vi "Create Event.vi"(8 "error in":errorcluster, 11 "SEQ in":refnum<class "SEQ.lvclass">) -> (0 "error out":errorcluster, 2 "MSG Event Reg":refnum<event-registration>, 3 "SEQ out":refnum<class "SEQ.lvclass">)   [LabVIEW 2014]
uses:
  SEQ.lvclass
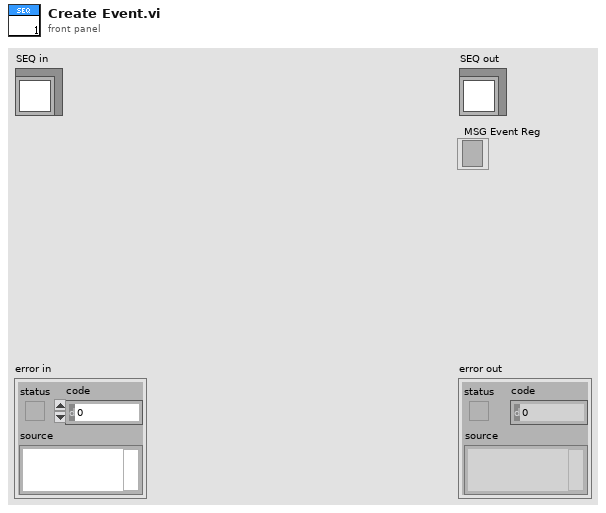
[diagram p1: front panel]
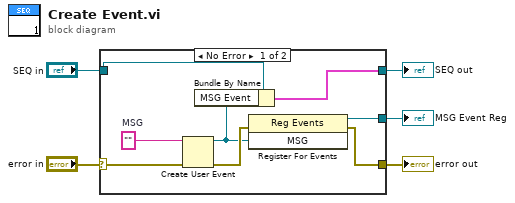
[diagram p0: block diagram]
diagram:
  n1 = case shown="No Error" "error in" {
    selector: "error in" -> [w12 w15]
    tunnel: [w10 w15] -> w4
    tunnel: [w6 w14] -> w2
    tunnel: "SEQ in" -> [w9 w14]
    tunnel: [w7 _] -> w1
    frame No Error {
      w13 = ""  # MSG
      n2 = Create User Event(user event datatype=w13, error in=w12) -> (user event=w8:refnum<user-event>, error out=w11:errorcluster)
      n3 = Bundle By Name(cluster=w9, "MSG Event"=w8) -> (w6:cluster{})
      n4 = register-events(error in=w11, w8) -> (reference out=w7:refnum<event-registration>, error out=w10:errorcluster)  [unwired: 1 in]
    }
    frame Error {
    }
  }
  "error out" <- w4
  "SEQ out" <- w2
  "MSG Event Reg" <- w1
